vi "Main modul map v3 GPS + kinematyka 2.vi"() -> ()   [LabVIEW 2015]
uses:
  <vilib>/Utility/miscctls.llb/LVPoint32TypeDef.ctl
  Kontrolki/Parametry odwzorowania Ziemi.ctl
  <vilib>/Utility/miscctls.llb/LVBoundsTypeDef.ctl
  <vilib>/Utility/miscctls.llb/LVPointTypeDef.ctl
  <vilib>/Utility/file.llb/Read From Spreadsheet File (string).vi
  Zmienne/szablon odometry_filtered_local.vi
  <vilib>/regexp/Match Regular Expression.xnode
  Pomocnicze/Pomocnicze.lvlib
  Zmienne/Zmienne.lvlib
  Matematyczne/Matematyczne.lvlib
  Kontrolki/Kontrolki.lvlib
panel:
  out "Lokalizacja robotów 2":T1
  in  "stop":bool
  out "Odl. pkt. od startu":cluster{"E/x[m]":dbl, "N/y[m]":dbl}
  out "Numeric":i32
  out "Obr. doj. do pkt.":timestamp
  out "x-y":u32
  in  "Poł. X.":T2={"UTM"={"E [m]"=276177.7293177693, "N [m]"=1172675.379150019, "Strefa"="38P"}, "Piksele"={"X"=991, "Y"=338}} {"UTM"."N [m]" format="%#_10g"}
  out "Mapa":picture caption="Mapa z wprowadzonym punktem"
  out "Lista współrzędnych":string[][](table)
  in  "Tab Control":T3(tab)
  in  "Azymut robota\n pocz/nowy":dbl caption="Azymut robota pocz/nowy" min=0.0 max=360.0
  in  "Lokalizacja mapy terenu":path=path "C:/Users/User/Desktop/Łazik/Mapy do ERL/zoom 19 szarosc - przycieta.jpg"
  in  "Parametry odwzorowania\n Ziemi (WGS84)":T4={"a"=6378137.0, "b"=6356752.3142} {"b" format="%#.6g"; "a" format="%#.6g"}
  in  "Lok. mapy odświeżanej":path=path "C:/Users/User/Desktop/Łazik/Zapis zebranych danych/zapis przejazdu.JPG" caption="Autozapis  mapy terenu"
  in  "Punkt o znanych współrzędnych (X)":T5={"Długość geograficzna - GPS"=10.601698, "Szerokośc geograficzna - GPS"=42.954275} {"Szerokośc geograficzna - GPS" format="%_9f"; "Długość geograficzna - GPS" format="%_9f"}
  in  "Ustawienia początkowe":T6={"Dane z"=TRUE, "Odometria z ROS'a"=TRUE, "GPS"=TRUE, "IMU"=TRUE}
  in  "Zapis danych z przejazdu":T7={"Łazik"=path "C:/Users/User/Desktop/Łazik/Zapis zebranych danych/Łazik.txt", "Quadron"=path "C:/Users/User/Desktop/Łazik/Zapis zebranych danych/Quadron.txt", "Dron 1"=path "C:/Users/User/Desktop/Łazik/Zapis zebranych danych/Dron 1.txt", "Dron 2"=path "C:/Users/User/Desktop/Łazik/Zapis zebranych danych/Dron 2.txt", "Sparus"=path "C:/Users/User/Desktop/Łazik/Zapis zebranych danych/Sparus.txt"}
  in  "Poł. start. robota":bool
  in  "Poł. start. wzgl. bazy":bool
  in  "Zakres skali":u16(ring)=11 items=["OSM 10m", "OSM 30m", "OSM 50m", "OSM 100m", "Google 10m", "Google 50m", "Google 200m1", "Google 100m", "Google 200m 2", "Google 500m", "Google zoom 17", "google zoom 18", "Google zoom 19"]
  in  "Skalowanie":T8={"Polozenie 1"={"X"=265, "Y"=265}, "  Wybór \nznacznika"=FALSE, "   Polozenie 2"={"X"=358, "Y"=265}, "   Blokada \nznaczników"=TRUE, "Kolor  znaczników"=16774930, "Grubość \nznaczników"=2, "Wyznaczanie odległości"=enum."Odległość pomiędzy znacznikami", "Współrzędne geograficzne 1"="", "Współrzędne geograficzne 2"="", "Odl. pomiędzy znacznikami [m]"=15.0}
  in  "Zatwierdz ustalony zakres":bool
  in  "Nazwa akt. pkt":string
  in  "Wpr. pkt. wsp. z pliku":bool
  in  "Plik z punktami wsp. geograficzne":path=path "C:/Users/User/Desktop/ERL 2017/GC.txt"
  in  "Obsługa punktów":T9 {"Usuń punkt z listy"."Punkt do usunięcia" items=["X"=1, "1G"=2, "2G"=3, "3G"=4, "4G"=5, "5G"=6, "6G"=7, "1A"=8, "2A"=9, "3A"=10]}
  in  "Dodaj pkt. poł robota":bool
  in  "Dodaj punkt przed docelowym":u16(ring) items=["X"=1, "1G"=2, "2G"=3, "3G"=4, "4G"=5, "5G"=6, "6G"=7, "1A"=8, "2A"=9, "3A"=10]
  out "Osiągnięcie punktu":bool caption="WP reached"
  out "Punkt\n docelowy":string caption="Punkt  aktualny"
  in  "jazda":bool caption="1. Jazda"
  in  "zad. promien \nodlegl. [m]":dbl=0.3
  in  "2. Autonomia":bool
  in  "Punkt  startowy":u16(ring) items=["X"=1, "1G"=2, "2G"=3, "3G"=4, "4G"=5, "5G"=6, "6G"=7, "1A"=8, "2A"=9, "3A"=10]
  in  "go forward":bool caption="Go forward"
  in  "Time to wait [s]":dbl
  in  "button/time":bool
  in  "Parametry regulatora":cluster{"kp":dbl, "k alfa":dbl, "k beta":dbl}={"kp"=0.2, "k alfa"=0.3, "k beta"=-0.02}
  in  "Dodaj punkt odl.":bool
  in  "Reset":T10
  in  "Wyczyść trasę":bool
  in  "Właściwości mapy":T12={"Przesunięcie mapy"={"X"=0, "Y"=0}, "Dł. px[m]"=0.19634281539316645, "Zoom mapy"=1.0, "Wpisane punkty na\nliście współrzędnych"=1638620, "Zaznaczony punkt"=14417920, "Układ współrzędnych"=786176, "Początkowe położenie robota"=16777215, "Trasa robota - Łazik"=2815743, "Ost. zazn. pkt"={"X"=0, "Y"=0}, "Draw Area Size"={"Width"=528, "Height"=564}} {"Zoom mapy" scale=0.2..6.0}
  out "V - prędkość postępowa":dbl(graph)
  out "w - prędkość kątowa":dbl(graph)
  in  "Wybór robota 3":T13 items=["Łazik", "Quadron", "Dron 1", "Dron 2", "Sparus"]
  in  "Wybór robota 2":T13 items=["Łazik", "Quadron", "Dron 1", "Dron 2", "Sparus"]
  out "Odległości pomiędzy wybranymi robotami xy [m]":cluster{"X [m]":dbl, "Y [m]":dbl}
  out "Odległość pomiędzy\n robotami [m]":dbl
  in  "Wybór robota":T13 items=["Łazik", "Quadron", "Dron 1", "Dron 2", "Sparus"]
  out "Odległość robota  \nod bazy  [m]":cluster{"X [m]":dbl, "Y [m]":dbl}
  out "Azymut":dbl(knob) scale=0.0..360.0
  out "Odczyt GPS":T14 caption="Położenie wybranego robota" {"Szerokośc geograficzna \n- GPS" format="%_9f"; "Długość geograficzna \n- GPS" format="%_9f"; "Położenie \nrobota  UTM"."E [m]" format="%#_10g"; "Położenie \nrobota  UTM"."N [m]" format="%#_12g"}
  in  "Legenda":T15={"Raptor"=16318208, "Quadron"=16711680, "Dron 1"=16777215, "Dron 2"=39423, "Sparus"=6618880}
  in  "Centr. Położenie robota":bool
  in  "Mouse down":T16
  # "Format wprowadzanych współrzędnych:\n0.0d N 0.0d E\n0.0d E 0.0d N\n0d 0.0m N 0d 0.0m E\n0d 0.0m E 0d 0.0m N\n0d 0m 0.0s N 0d 0m 0.0s E\n0d 0m 0.0s E 0d 0m 0.0s N\n\n\"0\" - oznacza dowolny ciąg cyfr. W miejscach gdzie występują liczby\ndziesiętne części całkowite od dziesiętnych są oddzielone znakiem\nkropki \".\".\nd - symbol stopni\nm - symbol minut\ns - symbol sekund\nN - symbol północnej szerokości geograficznej. Dla szerokości geograficznej południowej należy zastosować znak \"S\".\nE - symbol wschodniej długości geograficznej. Dla zachodniej długości geograficznej należy zastosować znak \"W\"."
  # "Nie można usuwać \npunktów, gdy włączona \njest autonomia"
  # "Robot zatrzyma się w najbliższym punkcie,\n który nie zawiera w nazwie litery P"
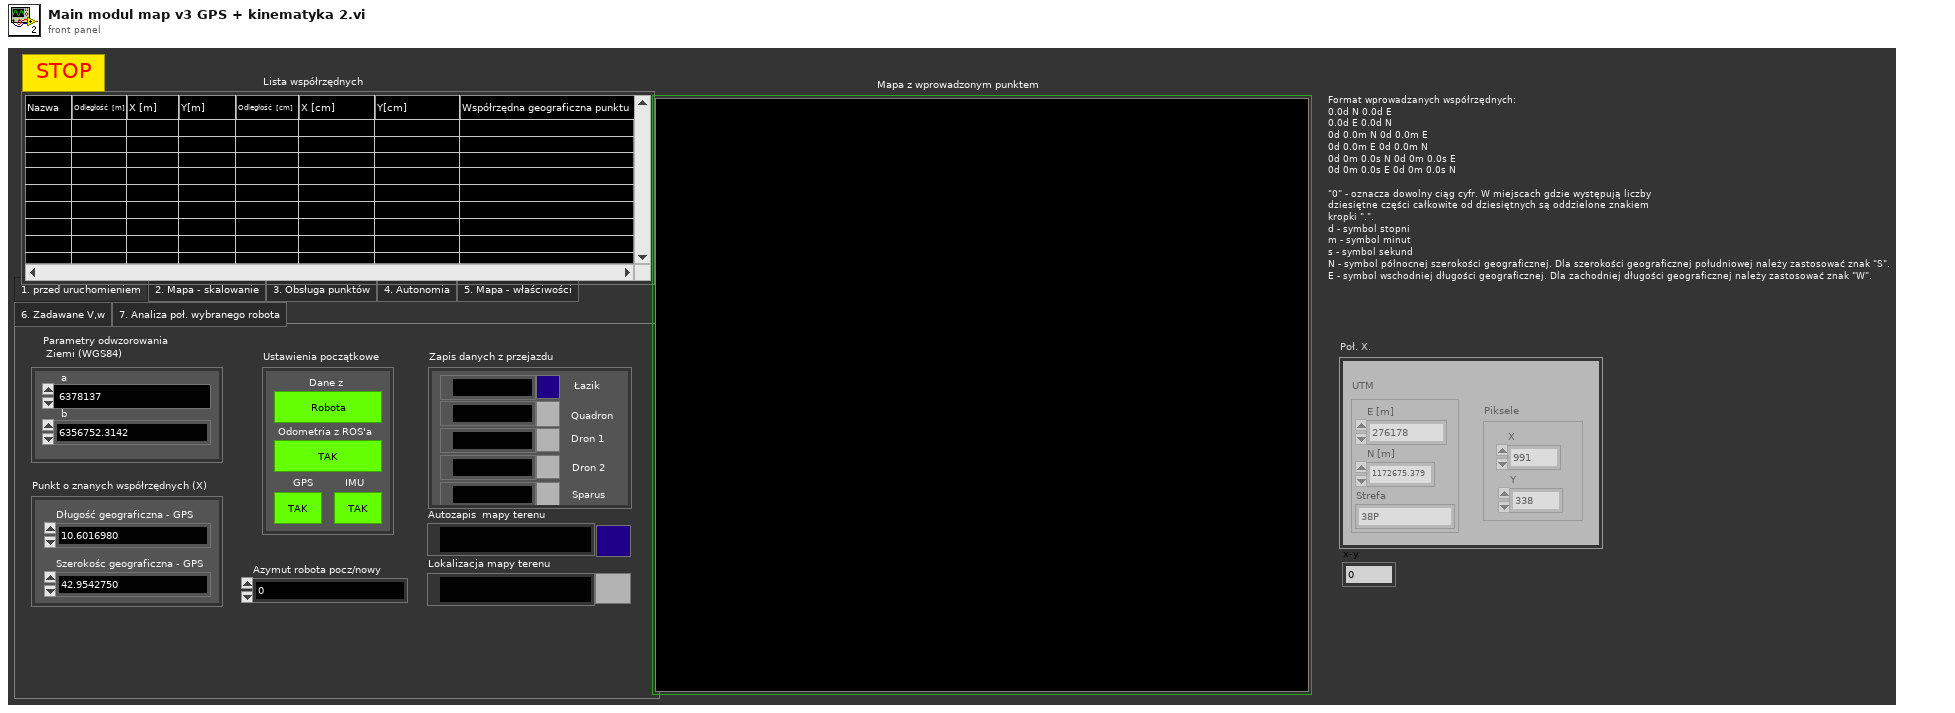
[diagram p1: front panel]
types:
  T1 = typedef "Biblioteka moduł map v3.lvlib/Kontrolki.lvlib/Lokalizacja robotów.ctl" = cluster{"Łazik":cluster{"Odczyt GPS":cluster{"Położenie \nrobota  UTM":cluster{"E [m]":ext, "N [m]":ext, "Strefa":string}, "Długość geograficzna - GPS":dbl, "Szerokośc geograficzna - GPS":dbl, "Azymut [stopnie]":dbl}, "Rzeczywista odległość\n robota od X [m]":cluster{"X [m]":dbl, "Y [m]":dbl}}, "Quadron":cluster{"Odczyt GPS":cluster{"Położenie \nrobota  UTM":cluster{"E [m]":ext, "N [m]":ext, "Strefa":string}, "Długość geograficzna - GPS":dbl, "Szerokośc geograficzna - GPS":dbl, "Azymut [stopnie]":dbl}, "Rzeczywista odległość\n robota od X [m]":cluster{"X [m]":dbl, "Y [m]":dbl}}, "Dron 1":cluster{"Odczyt GPS":cluster{"Położenie \nrobota  UTM":cluster{"E [m]":ext, "N [m]":ext, "Strefa":string}, "Długość geograficzna - GPS":dbl, "Szerokośc geograficzna - GPS":dbl, "Azymut [stopnie]":dbl}, "Rzeczywista odległość\n robota od X [m]":cluster{"X [m]":dbl, "Y [m]":dbl}}, "Dron 2":cluster{"Odczyt GPS":cluster{"Położenie \nrobota  UTM":cluster{"E [m]":ext, "N [m]":ext, "Strefa":string}, "Długość geograficzna - GPS":dbl, "Szerokośc geograficzna - GPS":dbl, "Azymut [stopnie]":dbl}, "Rzeczywista odległość\n robota od X [m]":cluster{"X [m]":dbl, "Y [m]":dbl}}, "Sparus":cluster{"Odczyt GPS":cluster{"Położenie \nrobota  UTM":cluster{"E [m]":ext, "N [m]":ext, "Strefa":string}, "Długość geograficzna - GPS":dbl, "Szerokośc geograficzna - GPS":dbl, "Azymut [stopnie]":dbl}, "Rzeczywista odległość\n robota od X [m]":cluster{"X [m]":dbl, "Y [m]":dbl}}}
  T2 = cluster{"UTM":cluster{"E [m]":dbl, "N [m]":dbl, "Strefa":string}, "Piksele":cluster{"X":i32, "Y":i32}}
  T3 = enum32{"1. przed uruchomieniem", "2. Mapa - skalowanie", "3. Obsługa punktów", "4. Autonomia", "5. Mapa - właściwości", "6. Zadawane V,w", "7. Analiza poł. wybranego robota"}
  T4 = typedef "Biblioteka moduł map v3.lvlib/Kontrolki.lvlib/Parametry odwzorowania Ziemi.ctl" = cluster{"a":dbl, "b":dbl}
  T5 = cluster{"Długość geograficzna - GPS":dbl, "Szerokośc geograficzna - GPS":dbl}
  T6 = cluster{"Dane z":bool, "Odometria z ROS'a":bool, "GPS":bool, "IMU":bool}
  T7 = cluster{"Łazik":path, "Quadron":path, "Dron 1":path, "Dron 2":path, "Sparus":path}
  T8 = cluster{"Polozenie 1":cluster{"X":i32, "Y":i32}, "  Wybór \nznacznika":bool, "   Polozenie 2":cluster{"X":i32, "Y":i32}, "   Blokada \nznaczników":bool, "Kolor  znaczników":u32, "Grubość \nznaczników":u32, "Wyznaczanie odległości":enum16{"Współrzędne geograficzne", "Odległość pomiędzy znacznikami"}, "Współrzędne geograficzne 1":string, "Współrzędne geograficzne 2":string, "Odl. pomiędzy znacznikami [m]":dbl}
  T9 = cluster{"Zaznaczony punkt":cluster{"Nazwa":string, "Odl. do pkt [m]":cluster{"X":dbl, "Y":dbl}, "Dodaj punkt odl.":bool}, "Wsp. geograficzne":cluster{"Nazwa":string, "Współrzędna punktu":string, "Dodaj punkt wsp.":bool}, "Usuń punkt z listy":cluster{"Punkt do usunięcia":u16, "Usuń punkt":bool}}
  T10 = cluster{"reset odom":bool, "reset odom + gps":bool}
  T11 = typedef "LVBoundsTypeDef.ctl" = cluster{"Width":u32, "Height":u32}
  T12 = cluster{"Przesunięcie mapy":cluster{"X":i16, "Y":i16}, "Dł. px[m]":dbl, "Zoom mapy":sgl, "Wpisane punkty na\nliście współrzędnych":u32, "Zaznaczony punkt":u32, "Układ współrzędnych":u32, "Początkowe położenie robota":u32, "Trasa robota - Łazik":u32, "Ost. zazn. pkt":cluster{"X":i32, "Y":i32}, "Draw Area Size":T11}
  T13 = typedef "Biblioteka moduł map v3.lvlib/Kontrolki.lvlib/Wybór robota.ctl" = u16
  T14 = cluster{"Położenie \nrobota  UTM":cluster{"E [m]":ext, "N [m]":ext, "Strefa":string}, "Długość geograficzna \n- GPS":dbl, "Szerokośc geograficzna \n- GPS":dbl, "Azymut [stopnie]":dbl}
  T15 = cluster{"Raptor":u32, "Quadron":u32, "Dron 1":u32, "Dron 2":u32, "Sparus":u32}
  T16 = typedef "LVPoint32TypeDef.ctl" = cluster{"Horizontal":i32, "Vertical":i32}
  T17 = enum16{"Pobranie punktu", "Obrót i dojazd do punktu", "Zatrzymanie w punkcie"}
  T18 = cluster{"UTM":cluster{"E [m]":ext, "N [m]":ext, "Strefa":string}, "Piksele":cluster{"X":i32, "Y":i32}}
  T19 = typedef "Biblioteka moduł map v3.lvlib/Zmienne.lvlib/szablon odometry_filtered_local.ctl" = cluster{"topic":string, "msg":cluster{"header":cluster{"seq":u32, "stamp":cluster{"secs":u32, "nsecs":i32}, "frame_id":string}, "child_frame_id":string, "pose":cluster{"pose":cluster{"position":cluster{"y":dbl, "z":dbl, "x":dbl}, "orientation":cluster{"y":dbl, "z":dbl, "x":dbl, "w":dbl}}, "covariance":dbl[]}, "twist":cluster{"twist":cluster{"linear":cluster{"y":dbl, "z":dbl, "x":dbl}, "angular":cluster{"y":dbl, "z":dbl, "x":dbl}}, "covariance":dbl[]}}, "op":string}
  T20 = cluster{"left":i16, "top":i16, "right":i16, "bottom":i16}
  T21 = cluster{"Nazwa zaznaczonego punktu":string, "Odleglosc do\n zaznaczonego punktu [m]":cluster{"X":dbl, "Y":dbl}}
  T22 = cluster{"Kolor punktów z listy":u32, "Położenie startowe robota":cluster{"Pixel y":i16, "Pixel x":i16}}
  T23 = typedef "LVPointTypeDef.ctl" = cluster{"Horizontal":i16, "Vertical":i16}
  T24 = cluster{"E [m]":dbl, "N [m]":dbl, "Strefa":string}
  T25 = typedef "LVMouseTypeDef.ctl" = cluster{"Mouse Position":cluster{"X":i32, "Y":i32}, "Mouse Modifiers":cluster{"Button Down":bool, "Shift Mod":bool, "Menu Mod":bool, "Option Mod":bool}}
  T26 = cluster{"Przesunięcie mapy":cluster{"X":i16, "Y":i16}, "Długość piksela w metrach":dbl, "Zoom mapy":sgl, "Wpisane punkty na\nliście współrzędnych":u32, "Zaznaczony punkt":u32, "Układ współrzędnych":u32, "Początkowe położenie robota":u32, "Trasa robota":u32, "Ost. zazn. pkt.":cluster{"X":i32, "Y":i32}, "Draw Area Size":T11}
  T27 = cluster{"Zaznaczony punkt":cluster{"Nazwa":string, "Odleglosc do\n zaznaczonego punktu [m]":cluster{"X":dbl, "Y":dbl}, "Dodaj punkt odl.":bool}, "Wsp. geograficzne":cluster{"Nazwa":string, "Współrzędna punktu":string, "Dodaj punkt wsp.":bool}, "Usuń punkt z listy":cluster{"Punkt do usunięcia":u16, "Usuń punkt":bool}}
  T28 = cluster{"E [m]":ext, "N [m]":ext, "Strefa":string}
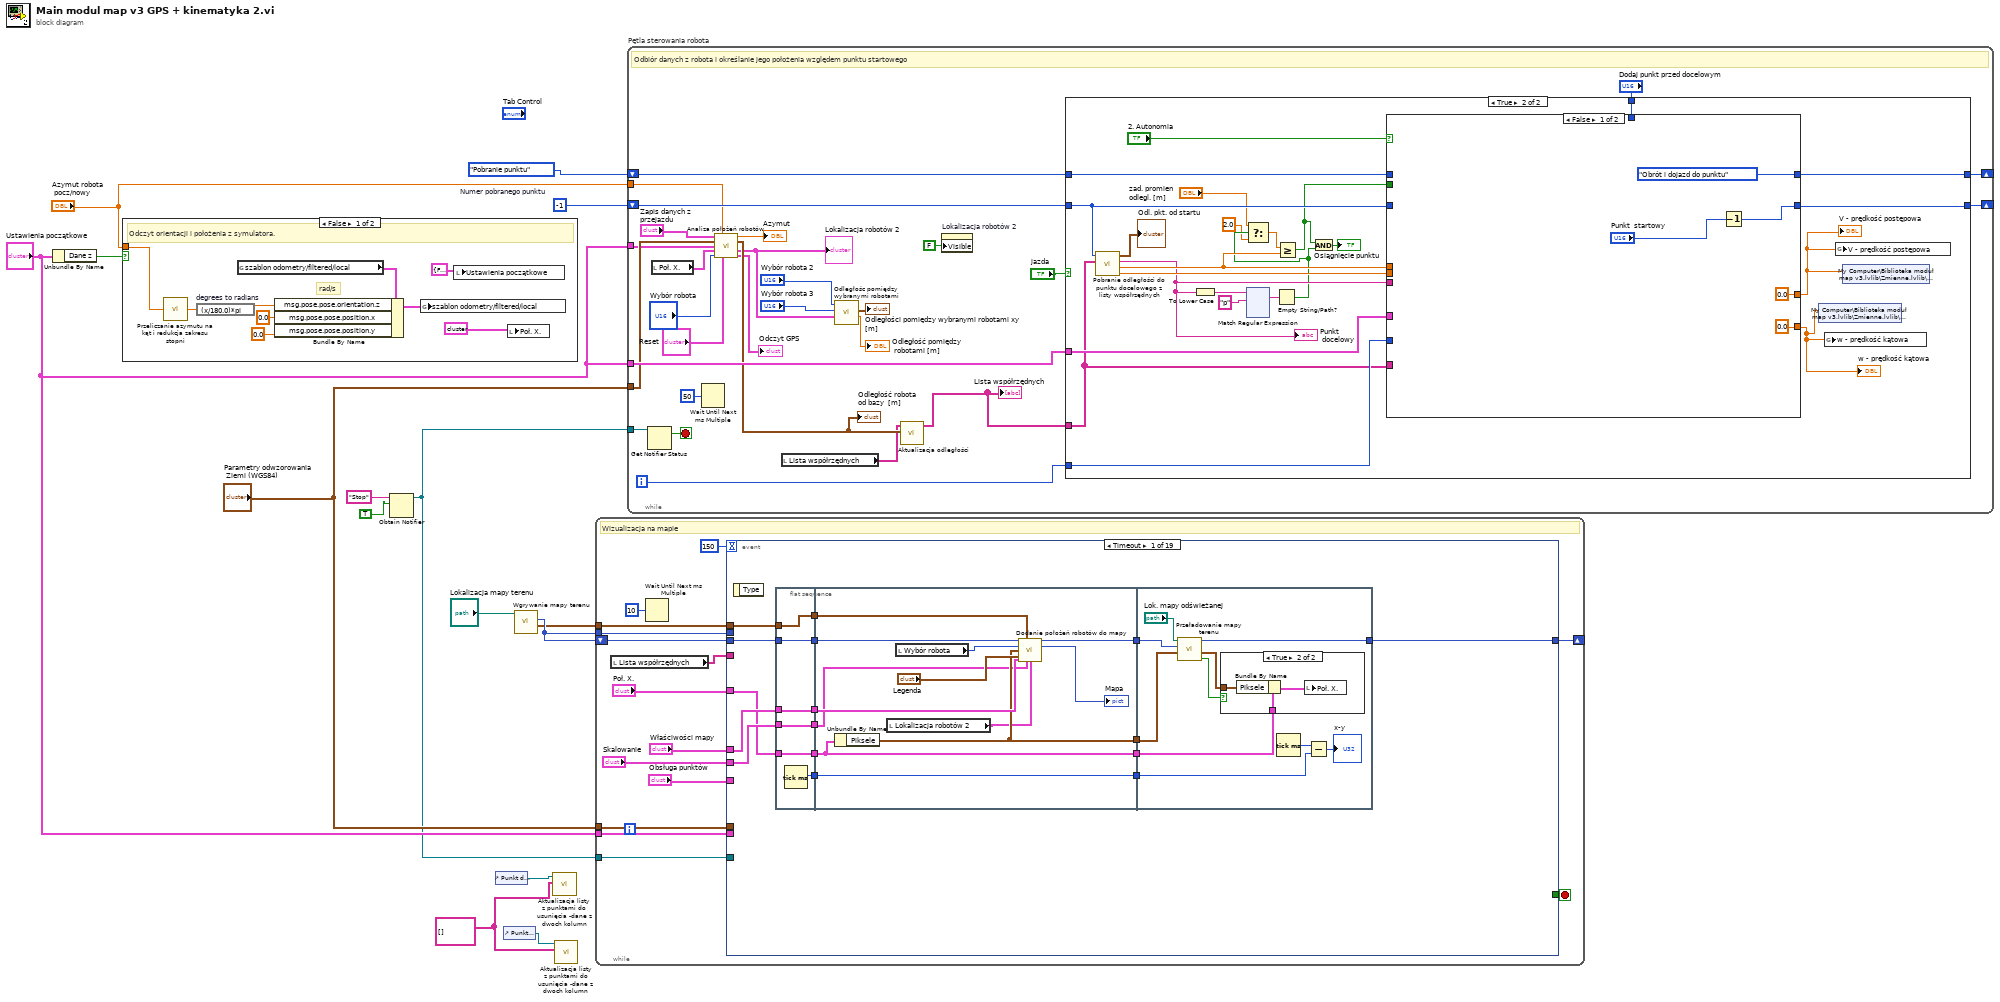
[diagram p0: block diagram]
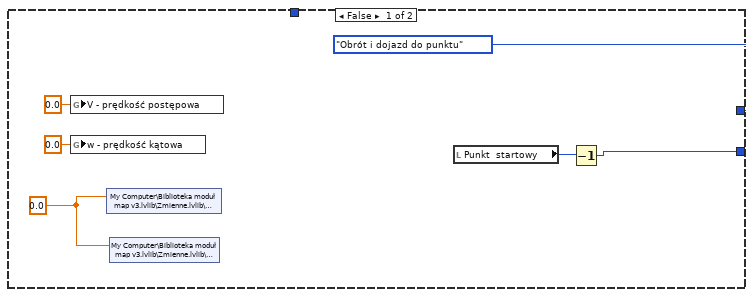
[diagram p3: hidden frame]
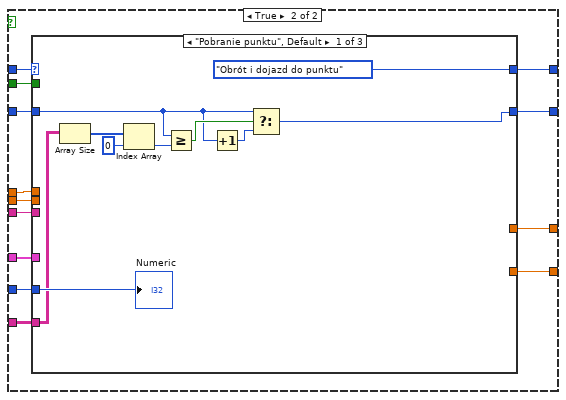
[diagram p4: hidden frame]
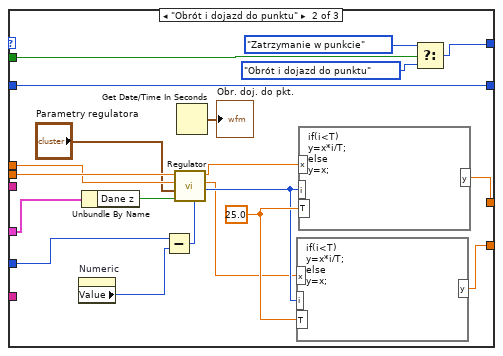
[diagram p5: hidden frame]
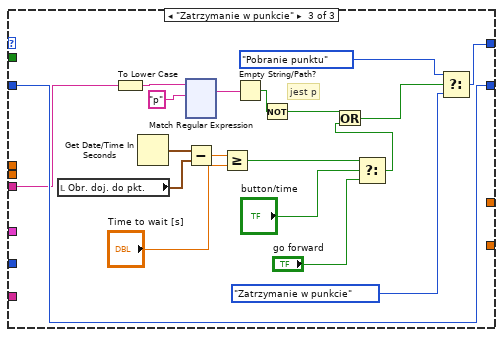
[diagram p6: hidden frame]
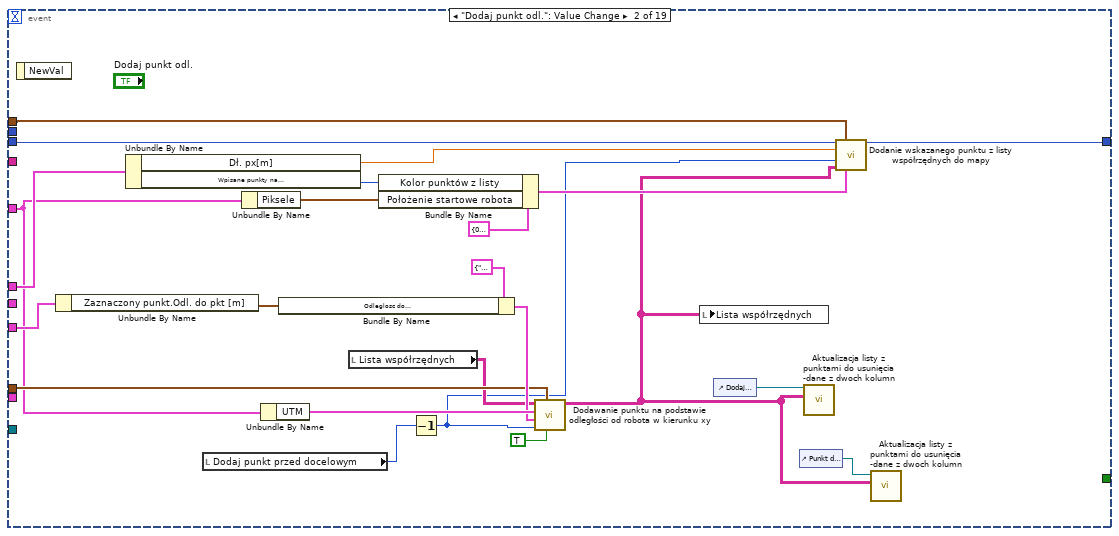
[diagram p8: hidden frame]
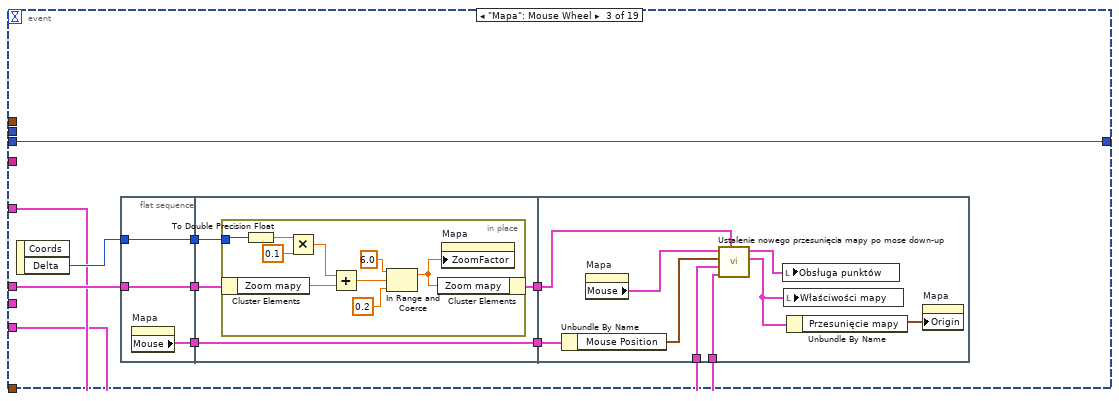
[diagram p9: hidden frame]
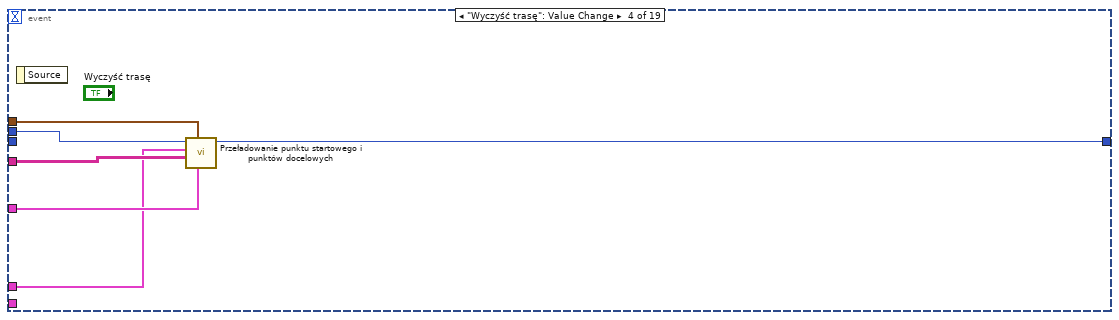
[diagram p10: hidden frame]
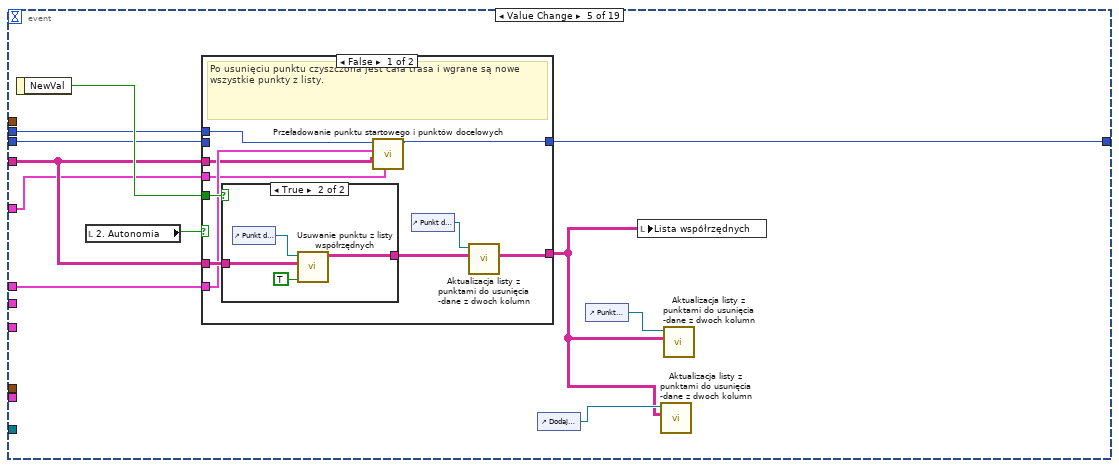
[diagram p11: hidden frame]
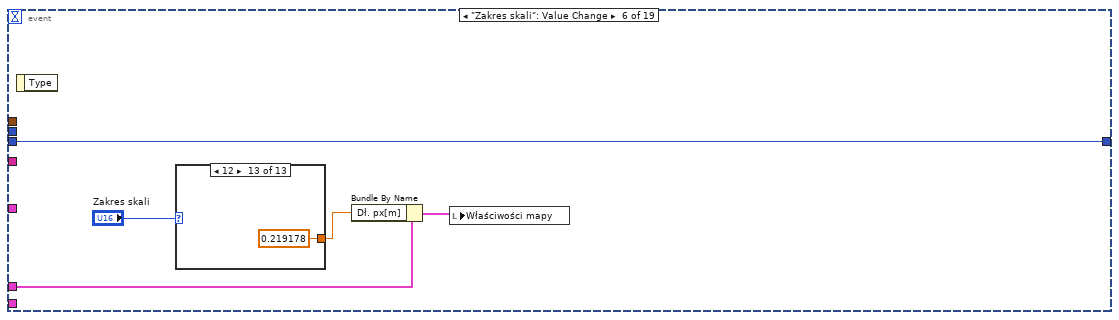
[diagram p14: hidden frame]
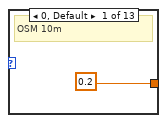
[diagram p15: hidden frame]
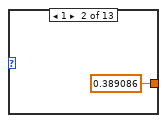
[diagram p16: hidden frame]
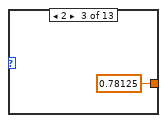
[diagram p17: hidden frame]
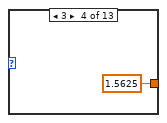
[diagram p18: hidden frame]
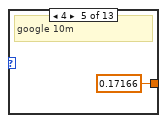
[diagram p19: hidden frame]
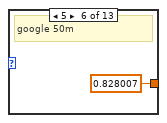
[diagram p20: hidden frame]
diagram:
  w5 = string[][] [] ("Lista współrzędnych")
  w14 = -1  # Numer pobranego punktu
  n1 = Unbundle By Name("Ustawienia początkowe") -> ("Dane z"=w4:bool)
  n2 = case shown="False" w4 {
    tunnel: "Azymut robota\n pocz/nowy" -> [w17 _]
    frame False {
      # "rad/s"
      # "Odczyt orientacji i położenia z symulatora."
      n3 = call "Przeliczanie azymutu na kąt i redukcja zakresu stopni.vi"("Azymut [stoponie]"=w17) -> ("Kąt [stopnie]"=w19:dbl)  [unwired: 4 in]
      n4 = expression code="(x/180.0)*pi" "degrees to radians"(w19) -> (w22:dbl)
      n5 = global read "szablon odometry_filtered_local.vi" "szablon odometry/filtered/local"() -> (w24:T19)
      n6 = Bundle By Name(cluster=w24, "msg.pose.pose.orientation.z"=w22, "msg.pose.pose.position.x"=0.0, "msg.pose.pose.position.y"=0.0) -> (w23:T19)
      n7 = global write "szablon odometry_filtered_local.vi" "szablon odometry/filtered/local"(w23) -> ()
      n8 = local write "Ustawienia początkowe"(T6 {"Dane z"=FALSE, "Odometria z ROS'a"=FALSE, "GPS"=FALSE, "IMU"=FALSE} ("Ustawienia początkowe")) -> ()
      n9 = local write "Poł. X."(T18 {"UTM"={"E [m]"=0.0, "N [m]"=0.0, "Strefa"=""}, "Piksele"={"X"=0, "Y"=0}} ("Pocz. bazowe.")) -> ()
    }
    frame True {
      # "Dane odczytywane z robota i zapisane w zmiennej globalnej."
    }
  }
  n10 = Obtain Notifier(name (unnamed)="Stop", notification data type=TRUE ("create if not found? (T)")) -> (notifier out=w1:refnum<notifier>)  [unwired: 2 in, 2 out]
  n11 = control-ref of="Punkt do usunięcia"() -> (w8:refnum<vi>)
  n12 = control-ref of="Punkt  startowy"() -> (w7:refnum<vi>)
  n13 = call "Wgrywanie mapy terenu.vi"("Lokalizacja mapy terenu"="Lokalizacja mapy terenu") -> ("Rozmiar mapy"=w6:T20, "Mapa terenu"=w12:picture)  [unwired: 9 in]
  n14 = call "Aktualizacja listy z punktami do usunięcia -dane z dwoch kolumn.vi"("Lista współrzędnych"=w5, "Lista z punktami do usunięcia"=w8) -> ()  [unwired: 10 in]
  n15 = call "Aktualizacja listy z punktami do usunięcia -dane z dwoch kolumn.vi"("Lista współrzędnych"=w5, "Lista z punktami do usunięcia"=w7) -> ()  [unwired: 10 in]
  n16 = while "Pętla obsługi mapy" {
    shift-right: [w36] -> _
    shift-left: w12 -> [w37]
    tunnel: "Parametry odwzorowania\n Ziemi (WGS84)" -> [w35]
    tunnel: w1 -> [w34]
    tunnel: w12 -> [w30]
    tunnel: w6 -> [w28]
    tunnel: "Ustawienia początkowe" -> [w27]
    stop <- w39 stop-if-true
    # "Wizualizacja na mapie"
    n17 = local read "Lista współrzędnych"() -> (w25:string[][])
    n18 = Wait Until Next ms Multiple(millisecond multiple=u32 10) -> ()  [unwired: 1 out]
    n19 = event shown="[0] Timeout" {
      selector: _ -> [_ _ _ _ _ _ _ _ _ _ _ _ _ _ _ _ _ _ _]
      dyn-events: _ -> [_ _ _ _ _ _ _ _ _ _ _ _ _ _ _ _ _ _ _]
      timeout: 150 -> [_ _ _ _ _ _ _ _ _ _ _ _ _ _ _ _ _ _ _]
      tunnel: "Właściwości mapy" -> [w54 w102 w117 w146 w155 w181 w213 w280 w292 w298 w315 w330 w351 w369 _ w386 w404 w430 w451]
      tunnel: w37 -> [w52 w103 w119 _ w157 w182 w216 w274 _ _ w321 w331 _ w371 w374 w387 w401 w437 w446]
      tunnel: [_ _ _ _ _ _ _ _ _ _ _ _ _ w365 _ _ _ _ _] -> w39
      tunnel: [w51 w101 w119 w150 w158 w182 w215 w272 w288 w299 w321 w331 w352 w371 w374 w387 w405 w437 w443] -> w36
      tunnel: w25 -> [_ _ _ w147 w154 _ w202 w282 w289 w301 _ _ w356 _ _ _ w408 _ w460]
      tunnel: w35 -> [_ w95 _ _ _ _ _ w285 _ w303 _ _ _ _ _ _ _ _ _]
      tunnel: w34 -> [_ _ _ _ _ _ _ _ _ _ _ _ _ w370 _ _ _ _ _]
      tunnel: "Poł. X." -> [w50 w94 w113 w148 w153 _ w209 w271 w286 _ _ w327 w344 _ _ w375 w403 w423 w442]
      tunnel: "Skalowanie" -> [w53 _ _ _ _ _ _ _ w295 _ _ _ _ _ _ w377 _ _ _]
      tunnel: "Obsługa punktów" -> [_ w96 w112 _ _ _ _ w283 _ _ _ _ _ _ _ w384 _ w426 w455]
      tunnel: w30 -> [_ _ _ w149 w156 _ _ _ w291 w302 _ _ w355 _ _ _ _ _ _]
      tunnel: w28 -> [w41 w104 _ w145 _ _ w214 w269 w287 w297 _ w323 w350 _ _ _ w400 _ w440]
      tunnel: w27 -> [_ _ _ _ _ _ w199 _ _ w300 _ _ w354 _ _ _ _ _ _]
      event Timeout {
        n20 = event-data() -> ()  [unwired: 1 in, 1 out]
        n21 = flat-sequence {
          tunnel: w50 -> [w58]
          tunnel: w52 -> [w59]
          tunnel: w53 -> [w60]
          tunnel: w54 -> [w61]
          tunnel: [w61] -> w47
          tunnel: [w60] -> w46
          tunnel: [w59] -> w45
          tunnel: [w58] -> w44
          tunnel: [w57] -> w43
          tunnel: w41 -> [w56]
          tunnel: [w56] -> w40
          tunnel: [w70] -> w55
          tunnel: [w64] -> w49
          tunnel: [w73] -> w48
          tunnel: w47 -> [w65]
          tunnel: w46 -> [w62]
          tunnel: w45 -> [w69]
          tunnel: w44 -> [w73]
          tunnel: w43 -> [w72]
          tunnel: [w72] -> w42
          tunnel: w40 -> [w68]
          tunnel: [w83] -> w51
          tunnel: w55 -> [w82]
          tunnel: w49 -> [w74]
          tunnel: w48 -> [w78]
          tunnel: w42 -> [w76]
          frame #0 {
            n22 = Tick Count (ms)() -> (millisecond timer value=w57:u32)
          }
          frame #1 {
            n23 = Unbundle By Name(w73) -> ("Piksele"=w64:cluster{"X":i32, "Y":i32})
            n24 = local read "Lokalizacja robotów 2"() -> (w63:T1)
            n25 = local read "Wybór robota"() -> (w67:T13)
            n26 = call "Dodanie położeń robotów do mapy.vi"("Mapa terenu"=w69, "Rozmiar mapy"=w68, "Wybór robota"=w67, "Poł. bazowe\n piksele"=w64, "Właściwości mapy"=w65, "Skalowanie i kolory"=w62, "Lokalizacja robotów"=w63, "Legenda"="Legenda") -> ("Mapa terenu stała"=w70:picture, "Mapa terenu wyświetlana"=→"Mapa":picture)  [unwired: 6 in]
          }
          frame #2 {
            n27 = call "Przeładowanie mapy terenu.vi"("Położenie startowe"=w74, ">mapa z trasą robota>"=w82, "path to JPEG file"="Lok. mapy odświeżanej") -> ("reload"=w81:bool, "Nowe położenie  startowe [px]"=w79:cluster{"X [px]":i16, "Y [px]":i16}, "Mapa terenu"=w83:picture)  [unwired: 6 in]
            n28 = case shown="True" w81 {
              tunnel: w79 -> [_ w86]
              tunnel: w78 -> [_ w85]
              frame False {
              }
              frame True {
                n29 = Bundle By Name(cluster=w85, "Piksele"=w86) -> (w84:T2)
                n30 = local write "Poł. X."(w84) -> ()
              }
            }
            n31 = Tick Count (ms)() -> (millisecond timer value=w77:u32)
            n32 = Subtract(x=w77, y=w76) -> (x-y=→"x-y":u32)
          }
        }
      }
      event "Dodaj punkt odl.": Value Change {
        n33 = event-data() -> ()  [unwired: 1 in, 1 out]
        n34 = Unbundle By Name(w96) -> ("Zaznaczony punkt.Odl. do pkt [m]"=w100:cluster{"X":dbl, "Y":dbl})
        n35 = Unbundle By Name(w102) -> ("Dł. px[m]"=w107:dbl, "Wpisane punkty na\nliście współrzędnych"=w108:u32)
        n36 = local read "Dodaj punkt przed docelowym"() -> (w88:u16)
        n37 = Unbundle By Name(w94) -> ("Piksele"=w105:cluster{"X":i32, "Y":i32})
        n38 = Unbundle By Name(w94) -> ("UTM"=w99:T24)
        n39 = Bundle By Name(cluster=T21 {"Nazwa zaznaczonego punktu"="p ", "Odleglosc do\n zaznaczonego punktu [m]"={"X"=23.89186471933565, "Y"=43.80175198544869}} ("Zaznaczony punkt"), "Odleglosc do\n zaznaczonego punktu [m]"=w100) -> (w98:T21)
        n40 = local read "Lista współrzędnych"() -> (w89:string[][])
        n41 = Bundle By Name(cluster=T22 {"Kolor punktów z listy"=0, "Położenie startowe robota"={"Pixel y"=0, "Pixel x"=0}} ("Właściwości punktów z listy"), "Kolor punktów z listy"=w108, "Położenie startowe robota"=w105) -> (w106:T22)
        n42 = Decrement(x=w88) -> (x-1=w87:u16)
        n43 = call "Dodawanie punktu na podstawie odległości od robota w kierunku xy.vi"("dodanie posredniego punktu w trybie autonomi"=TRUE, "Parametry odwzorowania Ziemi"=w95, "Nr wiersza do wpisania punktu"=w87, "Zaznaczony punkt"=w98, "Początkowe UTM"=w99, "Lista współrzędnych"=w89) -> ("output array"=w90:string[][])  [unwired: 5 in]
        n44 = local write "Lista współrzędnych"(w90) -> ()
        n45 = control-ref of="Dodaj punkt przed docelowym"() -> (w91:refnum<vi>)
        n46 = control-ref of="Punkt do usunięcia"() -> (w92:refnum<vi>)
        n47 = call "Aktualizacja listy z punktami do usunięcia -dane z dwoch kolumn.vi"("Lista współrzędnych"=w90, "Lista z punktami do usunięcia"=w91) -> ()  [unwired: 10 in]
        n48 = call "Dodanie wskazanego punktu z listy współrzędnych do mapy.vi"("Mapa terenu"=w103, "Rozmiar mapy"=w104, "Długość piksela w metrach"=w107, "Nr punktu"=w87, "Lista współrzędnych"=w90, "Właściwości punktów z listy"=w106) -> ("Mapa z wprowadzonym punktem"=w101:picture)  [unwired: 9 in]
        n49 = call "Aktualizacja listy z punktami do usunięcia -dane z dwoch kolumn.vi"("Lista współrzędnych"=w90, "Lista z punktami do usunięcia"=w92) -> ()  [unwired: 10 in]
      }
      event "Mapa": Mouse Wheel {
        n50 = event-data() -> ("Delta"=w118:i32)  [unwired: 1 in, 1 out]
        n51 = flat-sequence {
          tunnel: w117 -> [w121]
          tunnel: w118 -> [w122]
          tunnel: [w122] -> w116
          tunnel: [w121] -> w115
          tunnel: [w120] -> w111
          tunnel: w116 -> [w126]
          tunnel: w115 -> [w125]
          tunnel: [w124] -> w114
          tunnel: w111 -> [w123]
          tunnel: [w123] -> w110
          tunnel: w114 -> [w137]
          tunnel: w113 -> [w140]
          tunnel: w112 -> [w139]
          tunnel: w110 -> [w136]
          frame #0 {
            n52 = property on="Mapa" class="Pict"() -> ("Mouse"=w120:T25)  [unwired: 2 in, 2 out]
          }
          frame #1 {
            n53 = in-place {
              in-place-border: w126 -> [w134]
              n54 = in-place-cluster #1(w125) -> ("Zoom mapy"=w131:sgl)
              n55 = To Double Precision Float(number=w134) -> (double precision float=w135:dbl)
              n56 = Multiply(x=w135, y=0.1) -> (x*y=w132:dbl)
              n57 = Add(x=w132, y=w131) -> (x+y=w130:dbl)
              n58 = In Range and Coerce(upper limit=6.0, x=w130, lower limit=0.2) -> (coerced(x)=w127:dbl)  [unwired: 1 out]
              n59 = in-place-cluster #1("Zoom mapy"=w127) -> (w124:T12)
              n60 = property on="Mapa" class="Pict"("ZoomFactor"=w127) -> ()  [unwired: 2 in, 2 out]
            }
          }
          frame #2 {
            n61 = Unbundle By Name(w136) -> ("Mouse Position"=w144:cluster{"X":i32, "Y":i32})
            n62 = property on="Mapa" class="Pict"() -> ("Mouse"=w138:T25)  [unwired: 2 in, 2 out]
            n63 = call "Ustalenie nowego przesunięcia mapy po mose down-up.vi"("Właściwości mapy in"=w137, "Pocz. poł."=w140, "Obsługa punktów in"=w139, "Mouse down \ncoords"=w144, "Mouse"=w138) -> ("Właściwości mapy out"=w142:T26, "Obsługa punktów out"=w141:T27)  [unwired: 5 in]
            n64 = local write "Obsługa punktów"(w141) -> ()
            n65 = local write "Właściwości mapy"(w142) -> ()
            n66 = Unbundle By Name(w142) -> ("Przesunięcie mapy"=w143:cluster{"X":i16, "Y":i16})
            n67 = property on="Mapa" class="Pict"("Origin"=w143) -> ()  [unwired: 2 in, 2 out]
          }
        }
      }
      event "Wyczyść trasę": Value Change {
        n68 = event-data() -> ()  [unwired: 1 in, 1 out]
        n69 = call "Przeładowanie punktu startowego i punktów docelowych.vi"("Pocz. poł. startu"=w148, "Rozmiar mapy"=w145, "Lista współrzędnych"=w147, "Właściwości mapy"=w146, "Mapa terenu"=w149) -> ("Mapa z wprowadzonym punktem"=w150:picture)  [unwired: 6 in]
      }
      event "Obsługa punktów.Usuń punkt z listy.Usuń punkt": Value Change {
        n70 = event-data() -> ("NewVal"=w161:bool)  [unwired: 1 in]
        n71 = local read "2. Autonomia"() -> (w160:bool)
        n72 = case shown="False" w160 {
          tunnel: w161 -> [w170 _]
          tunnel: w154 -> [w168 w177]
          tunnel: [w167 w177] -> w151
          tunnel: w157 -> [_ w176]
          tunnel: [w166 w176] -> w158
          tunnel: w156 -> [w165 _]
          tunnel: w155 -> [w164 _]
          tunnel: w154 -> [w163 _]
          tunnel: w153 -> [w162 _]
          frame False {
            # "Po usunięciu punktu czyszczona jest cała trasa i wgrane są nowe wszystkie punkty z listy."
            n73 = case shown="True" w170 {
              tunnel: w168 -> [w171 w174]
              tunnel: [w171 w173] -> w167
              frame False {
              }
              frame True {
                n74 = control-ref of="Punkt do usunięcia"() -> (w175:refnum<vi>)
                n75 = call "Usuwanie punktu z listy współrzędnych.vi"("Aktywacja potwierdzenia"=TRUE, "Lista współrzędnych"=w174, "Lista z punktami do usunięcia"=w175) -> ("Lista współrzędnych 2"=w173:string[][])  [unwired: 8 in]
              }
            }
            n76 = call "Przeładowanie punktu startowego i punktów docelowych.vi"("Pocz. poł. startu"=w162, "Lista współrzędnych"=w163, "Właściwości mapy"=w164, "Mapa terenu"=w165) -> ("Mapa z wprowadzonym punktem"=w166:picture)  [unwired: 7 in]
            n77 = control-ref of="Punkt do usunięcia"() -> (w169:refnum<vi>)
            n78 = call "Aktualizacja listy z punktami do usunięcia -dane z dwoch kolumn.vi"("Lista współrzędnych"=w167, "Lista z punktami do usunięcia"=w169) -> ()  [unwired: 10 in]
          }
          frame True {
          }
        }
        n79 = control-ref of="Dodaj punkt przed docelowym"() -> (w152:refnum<vi>)
        n80 = control-ref of="Punkt  startowy"() -> (w159:refnum<vi>)
        n81 = local write "Lista współrzędnych"(w151) -> ()
        n82 = call "Aktualizacja listy z punktami do usunięcia -dane z dwoch kolumn.vi"("Lista współrzędnych"=w151, "Lista z punktami do usunięcia"=w152) -> ()  [unwired: 10 in]
        n83 = call "Aktualizacja listy z punktami do usunięcia -dane z dwoch kolumn.vi"("Lista współrzędnych"=w151, "Lista z punktami do usunięcia"=w159) -> ()  [unwired: 10 in]
      }
      event "Zakres skali": Value Change {
        n84 = event-data() -> ()  [unwired: 1 in, 1 out]
        n85 = case shown="12" "Zakres skali" {
          tunnel: [0.2 0.389086 0.78125 1.5625 0.17166 0.828007 4.25179 3.81711 2.13015 8.47336 0.943026 0.471513 0.219178] -> w179
          frame 0, Default {
            # "OSM 10m"
          }
          frame 1 {
          }
          frame 2 {
          }
          frame 3 {
          }
          frame 4 {
            # "google 10m"
          }
          frame 5 {
            # "google 50m"
          }
          frame 6 {
            # "200m1"
          }
          frame 7 {
            # "100m"
          }
          frame 8 {
            # "200m2"
          }
          frame 9 {
            # "500m popr."
          }
          frame 10 {
            # "zoom 17 MPuzle"
          }
          frame 11 {
            # "18 zoom MP"
          }
          frame 12 {
          }
        }
        n86 = Bundle By Name(cluster=w181, "Dł. px[m]"=w179) -> (w180:T12)
        n87 = local write "Właściwości mapy"(w180) -> ()
      }
      event "Dodaj pkt. poł robota": Value Change {
        n88 = event-data() -> ()  [unwired: 1 in, 1 out]
        n89 = Unbundle By Name(w199) -> ("GPS"=w198:bool)
        n90 = Unbundle By Name(w209) -> ("Piksele"=w208:cluster{"X":i32, "Y":i32})
        n91 = Unbundle By Name(w213) -> ("Dł. px[m]"=w212:dbl, "Wpisane punkty na\nliście współrzędnych"=w207:u32)
        n92 = case shown="True" w198 {
          tunnel: [w237 w264] -> w196
          tunnel: w202 -> [w229 w263]
          tunnel: w209 -> [_ w262]
          tunnel: "Nazwa akt. pkt" -> [w222 w248]
          frame False {
            w224 = ""
            n93 = Array Size(array=w229) -> (size(s)=w235:i32[])
            n94 = local read "Odległość robota  \nod bazy  [m]"() -> (w217:cluster{"X [m]":dbl, "Y [m]":dbl})
            n95 = Index Array(array=w235, index=0) -> (element=w233:i32)
            n96 = Equal?(x=w222, y="Start") -> (x = y?=w221:bool)
            n97 = Increment(x=w233) -> (x+1=w232:i32)
            n98 = Number To Decimal String(number=w232) -> (decimal integer string=w230:string)  [unwired: 1 in]
            n99 = Empty String/Path?(string/path=w222) -> (empty?=w231:bool)
            n100 = Select(t=w230, s=w231, f=w222) -> (s? t:f=w220:string)
            n101 = Unbundle By Name(w217) -> ("X [m]"=w228:dbl, "Y [m]"=w227:dbl)
            n102 = Select(t="", s=w221, f=w220) -> (s? t:f=w219:string)
            n103 = Number To Fractional String(number=w228) -> (F-format string=w226:string)  [unwired: 3 in]
            n104 = Number To Fractional String(number=w227) -> (F-format string=w225:string)  [unwired: 3 in]
            n105 = Build Array(w219, w224, w224, w224, w224, w224, w224, w224, w224, w224, w224, w226, w225) -> (w236:string[])
            n106 = Insert Into Array(array=w229, new element=w236) -> (w237:string[][])  [unwired: 2 in]
          }
          frame True {
            n107 = local read "Odczyt GPS"() -> (w240:T14)
            n108 = Unbundle By Name(w262) -> ("UTM"=w261:T24)
            n109 = Unbundle By Name(w240) -> ("Długość geograficzna \n- GPS"=w239:dbl, "Szerokośc geograficzna \n- GPS"=w238:dbl)
            n110 = Greater Or Equal To 0?(x=w238) -> (x >= 0?=w258:bool)
            n111 = Absolute Value(x=w239) -> (abs(x)=w259:dbl)
            n112 = Greater Or Equal To 0?(x=w239) -> (x >= 0?=w257:bool)
            n113 = Absolute Value(x=w238) -> (abs(x)=w260:dbl)
            n114 = Number To Fractional String(number=w259) -> (F-format string=w252:string)  [unwired: 3 in]
            n115 = Select(t="d N " ("f"), s=w258, f="d S ") -> (s? t:f=w249:string)
            n116 = Number To Fractional String(number=w260) -> (F-format string=w250:string)  [unwired: 3 in]
            n117 = Select(t="d E " ("f"), s=w257, f="d W ") -> (s? t:f=w251:string)
            n118 = Concatenate Strings(w252, w251, w250, w249) -> (w247:string)
            n119 = Search and Replace String(input string=w247, search string=",", replace string="." ("replace string (\"\")")) -> (result string=w246:string)  [unwired: 5 in, 3 out]
            n120 = Search and Replace String(input string=w246, search string=",", replace string="." ("replace string (\"\")")) -> (result string=w245:string)  [unwired: 5 in, 3 out]
            n121 = call "Dodanie punktu do listy punkty na podstawie współrzędnych geograficznych.vi"("Nazwa punktu"=w248, "UTM"=w261, "Współrzędne punktu"=w245, "Lista wsp. in"=w263) -> ("Lista wsp. out"=w264:string[][])  [unwired: 7 in]
          }
        }
        n122 = Bundle By Name(cluster=T22 {"Kolor punktów z listy"=0, "Położenie startowe robota"={"Pixel y"=0, "Pixel x"=0}} ("Właściwości punktów z listy"), "Kolor punktów z listy"=w207, "Położenie startowe robota"=w208) -> (w205:T22)
        n123 = control-ref of="Dodaj punkt przed docelowym"() -> (w197:refnum<vi>)
        n124 = control-ref of="Punkt do usunięcia"() -> (w211:refnum<vi>)
        n125 = Array Size(array=w196) -> (size(s)=w203:i32[])
        n126 = Index Array(array=w203, index=0) -> (element=w201:i32)
        n127 = call "Aktualizacja listy z punktami do usunięcia -dane z dwoch kolumn.vi"("Lista współrzędnych"=w196, "Lista z punktami do usunięcia"=w197) -> ()  [unwired: 10 in]
        n128 = call "Aktualizacja listy z punktami do usunięcia -dane z dwoch kolumn.vi"("Lista współrzędnych"=w196, "Lista z punktami do usunięcia"=w211) -> ()  [unwired: 10 in]
        n129 = Decrement(x=w201) -> (x-1=w200:i32)
        n130 = local write "Lista współrzędnych"(w196) -> ()
        n131 = call "Dodanie wskazanego punktu z listy współrzędnych do mapy.vi"("Mapa terenu"=w216, "Rozmiar mapy"=w214, "Długość piksela w metrach"=w212, "Nr punktu"=w200, "Lista współrzędnych"=w196, "Właściwości punktów z listy"=w205) -> ("Mapa z wprowadzonym punktem"=w215:picture)  [unwired: 9 in]
      }
      event "Obsługa punktów.Zaznaczony punkt.Dodaj punkt odl.": Value Change {
        n132 = event-data() -> ()  [unwired: 1 in, 1 out]
        n133 = control-ref of="Punkt do usunięcia"() -> (w284:refnum<vi>)
        n134 = Unbundle By Name(w280) -> ("Dł. px[m]"=w276:dbl, "Wpisane punkty na\nliście współrzędnych"=w279:u32)
        n135 = call "Dodanie zaznaczonego punktu na podstawie odległości.vi"("output array in"=w282, "Pocz. poł."=w271, "Obsługa punktów"=w283, "Parametry odwzorowania Ziemi (WGS84)"=w285, "Ring in"=w284) -> ("output array out"=w265:string[][])  [unwired: 6 in]
        n136 = Unbundle By Name(w271) -> ("Piksele"=w273:cluster{"X":i32, "Y":i32})
        n137 = Bundle By Name(cluster=T22 {"Kolor punktów z listy"=0, "Położenie startowe robota"={"Pixel y"=0, "Pixel x"=0}} ("Właściwości punktów z listy"), "Kolor punktów z listy"=w279, "Położenie startowe robota"=w273) -> (w275:T22)
        n138 = Array Size(array=w265) -> (size(s)=w277:i32[])
        n139 = Index Array(array=w277, index=0) -> (element=w268:i32)
        n140 = Decrement(x=w268) -> (x-1=w267:i32)
        n141 = call "Dodanie wskazanego punktu z listy współrzędnych do mapy.vi"("Mapa terenu"=w274, "Rozmiar mapy"=w269, "Długość piksela w metrach"=w276, "Nr punktu"=w267, "Lista współrzędnych"=w265, "Właściwości punktów z listy"=w275) -> ("Mapa z wprowadzonym punktem"=w272:picture)  [unwired: 9 in]
        n142 = local write "Lista współrzędnych"(w265) -> ()
        n143 = control-ref of="Dodaj punkt przed docelowym"() -> (w266:refnum<vi>)
        n144 = control-ref of="Punkt  startowy"() -> (w270:refnum<vi>)
        n145 = call "Aktualizacja listy z punktami do usunięcia -dane z dwoch kolumn.vi"("Lista współrzędnych"=w265, "Lista z punktami do usunięcia"=w266) -> ()  [unwired: 10 in]
        n146 = call "Aktualizacja listy z punktami do usunięcia -dane z dwoch kolumn.vi"("Lista współrzędnych"=w265, "Lista z punktami do usunięcia"=w270) -> ()  [unwired: 10 in]
      }
      event "Zatwierdz ustalony zakres": Value Change {
        n147 = event-data() -> ()  [unwired: 1 in, 1 out]
        n148 = call "Zatwierdzenie ustalonego zakresu.vi"("Skalowanie in"=w295) -> ("Dł. piksela[m]"=w293:dbl, "Skalowanie out"=w294:T8)  [unwired: 9 in]
        n149 = local write "Skalowanie"(w294) -> ()
        n150 = Bundle By Name(cluster=w292, "Dł. px[m]"=w293) -> (w290:T12)
        n151 = local write "Właściwości mapy"(w290) -> ()
        n152 = call "Przeładowanie punktu startowego i punktów docelowych.vi"("Pocz. poł. startu"=w286, "Rozmiar mapy"=w287, "Lista współrzędnych"=w289, "Właściwości mapy"=w290, "Mapa terenu"=w291) -> ("Mapa z wprowadzonym punktem"=w288:picture)  [unwired: 6 in]
      }
      event "Poł. start. wzgl. bazy": Value Change {
        # "Ostatnie zaznaczone na mapie położenie odpowiada lokalizacji robota na mapie terenu."
        n153 = event-data() -> ()  [unwired: 1 in, 1 out]
        n154 = Unbundle By Name(w300) -> ("GPS"=w296:bool)
        n155 = case shown="True" w296 {
          tunnel: w303 -> [_ w309]
          tunnel: w302 -> [w304 w313]
          tunnel: w301 -> [_ w312]
          tunnel: [w304 w305] -> w299
          tunnel: w298 -> [_ w311]
          tunnel: w297 -> [_ w310]
          frame False {
          }
          frame True {
            # "Położenie startu robota na mapie określane na podstawie danych z GPS"
            n156 = local read "Mouse down"() -> (w308:T16)
            n157 = disable-structure shown="Disabled" {
              frame Disabled {
                n158 = local read "Odczyt GPS"() -> ()  [unwired: 1 out]
              }
              frame Enabled {
              }
            }
            n159 = call "Ustawienie startu względem punktu o znanych współrzędnych.vi"("Parametry odwzorowania\n Ziemi (WGS84)"=w309, "Punkt o znanych współrzędnych (baza)"="Punkt o znanych współrzędnych (X)", "Ost. zazn. punkt [px]"=w308) -> ("Poł. startu. out"=w306:T2)  [unwired: 8 in]
            n160 = call "Przeładowanie punktu startowego i punktów docelowych.vi"("Pocz. poł. startu"=w306, "Rozmiar mapy"=w310, "Lista współrzędnych"=w312, "Właściwości mapy"=w311, "Mapa terenu"=w313) -> ("Mapa z wprowadzonym punktem"=w305:picture)  [unwired: 6 in]
            n161 = local write "Poł. X."(w306) -> ()
          }
        }
      }
      event "Właściwości mapy.Zoom mapy": Value Change {
        n162 = event-data() -> ("NewVal"=w319:sgl)  [unwired: 1 in]
        n163 = local read "Mouse down"() -> (w314:T16)
        n164 = control-ref of="Mapa"() -> (w320:refnum<vi>)
        n165 = call "Centrowanie położenia.vi"("Ostatnie położenie robota"=w314, "Mapa z wprowadzonym punktem"=w320) -> ("Przesunięcie wycentrowane"=w317:T16)  [unwired: 9 in]
        n166 = Negate(x=w317) -> (-x=w316:T16)
        n167 = property on="Mapa" class="Pict"("Origin"=w316) -> ()  [unwired: 2 in, 2 out]
        n168 = Bundle By Name(cluster=w315, "Zoom mapy"=w319, "Przesunięcie mapy"=w316, "Ost. zazn. pkt"=w317) -> (w318:T12)
        n169 = property on="Mapa" class="Pict"("ZoomFactor"=w319) -> ()  [unwired: 2 in, 2 out]
        n170 = local write "Właściwości mapy"(w318) -> ()
      }
      event "Centr. Położenie robota": Value Change {
        n171 = event-data() -> ()  [unwired: 1 in, 1 out]
        n172 = local read "Odległość robota  \nod bazy  [m]"() -> (w325:cluster{"X [m]":dbl, "Y [m]":dbl})
        n173 = Unbundle By Name(w330) -> ("Dł. px[m]"=w329:dbl)
        n174 = Unbundle By Name(w327) -> ("Piksele"=w326:cluster{"X":i32, "Y":i32})
        n175 = in-place {
          in-place-border: w329 -> [w340]
          n176 = in-place-cluster #2(w325) -> ("X [m]"=w339:dbl, "Y [m]"=w338:dbl)
          n177 = Divide(x=w338, y=w340) -> (x/y=w341:dbl)
          n178 = Divide(x=w339, y=w340) -> (x/y=w343:dbl)
          n179 = Negate(x=w341) -> (-x=w342:dbl)
          n180 = in-place-cluster #2("X [m]"=w343, "Y [m]"=w342) -> (w328:cluster{"X [m]":dbl, "Y [m]":dbl})
        }
        n181 = Add(x=w328, y=w326) -> (x+y=w324:cluster{dbl, dbl})
        n182 = call "w zakresie mapy.vi"("Rozmiar mapy"=w323, "Poł. piksel"=w324) -> ("Boolean"=w322:bool)  [unwired: 9 in]
        n183 = case shown="True" w322 {
          tunnel: w330 -> [_ w333]
          tunnel: w324 -> [_ w332]
          frame False {
          }
          frame True {
            n184 = control-ref of="Mapa"() -> (w337:refnum<vi>)
            n185 = call "Centrowanie położenia.vi"("Ostatnie położenie robota"=w332, "Mapa z wprowadzonym punktem"=w337) -> ("Przesunięcie wycentrowane"=w335:T16)  [unwired: 9 in]
            n186 = Negate(x=w335) -> (-x=w334:T16)
            n187 = Bundle By Name(cluster=w333, "Przesunięcie mapy"=w334, "Ost. zazn. pkt"=w335) -> (w336:T12)
            n188 = property on="Mapa" class="Pict"("Origin"=w334) -> ()  [unwired: 2 in, 2 out]
            n189 = local write "Właściwości mapy"(w336) -> ()
          }
        }
      }
      event "Poł. start. robota": Value Change {
        # "Po wyborze poł. start. robota ostatni zaznaczony punkt na mapie staje się położenia m startowym."
        n190 = event-data() -> ()  [unwired: 1 in, 1 out]
        n191 = Unbundle By Name(w354) -> ("GPS"=w353:bool)
        n192 = Unbundle By Name(w351) -> ("Ost. zazn. pkt"=w349:cluster{"X":i32, "Y":i32})
        n193 = call "w zakresie mapy.vi"("Rozmiar mapy"=w350, "Poł. piksel"=w349) -> ("Boolean"=w348:bool)  [unwired: 9 in]
        n194 = Bundle By Name(cluster=w344, "Piksele"=w349) -> (w345:T2)
        n195 = Select(t=w345, s=w348, f=w344) -> (s? t:f=w347:T2)
        n196 = case shown="True" w353 {
          tunnel: w347 -> [w357 w359]
          tunnel: [w357 w358] -> w346
          frame False {
            # "Zapisanie do położenia startowego lokalizacji startu w pikselach bez uwzględnienia położenia GPS."
          }
          frame True {
            # "Zapisanie do położenia startowego lokalizacji startu w pikselach oraz dane GPS dla tego punktu."
            n197 = local read "Odczyt GPS"() -> (w361:T14)
            n198 = Unbundle By Name(w361) -> ("Położenie \nrobota  UTM"=w360:T28)
            n199 = Bundle By Name(cluster=w359, "UTM"=w360) -> (w358:T2)
          }
        }
        n200 = call "Przeładowanie punktu startowego i punktów docelowych.vi"("Pocz. poł. startu"=w346, "Rozmiar mapy"=w350, "Lista współrzędnych"=w356, "Właściwości mapy"=w351, "Mapa terenu"=w355) -> ("Mapa z wprowadzonym punktem"=w352:picture)  [unwired: 6 in]
        n201 = local write "Poł. X."(w346) -> ()
      }
      event "stop": Value Change {
        w366 = 0.0 ("V_postepowa")
        n202 = event-data() -> ()  [unwired: 1 in, 1 out]
        n203 = Bundle By Name(cluster=w369, "Przesunięcie mapy"=T23 {"Horizontal"=0, "Vertical"=0} ("Origin")) -> (w368:T12)
        n204 = shared-variable "My Computer\\Biblioteka moduł map v3.lvlib\\Zmienne.lvlib\\Predkosci robota.lvlib\\V_postepowa"(w366) -> ()  [unwired: 1 in, 1 out]
        n205 = shared-variable "My Computer\\Biblioteka moduł map v3.lvlib\\Zmienne.lvlib\\Predkosci robota.lvlib\\w-obrotowa"(w366) -> ()  [unwired: 1 in, 1 out]
        n206 = local write "Właściwości mapy"(w368) -> ()
        n207 = Two Button Dialog(message="Czy zakończyć działanie programu?", 1:"NIE" ("F button name (\"Cancel\")"), 2:"TAK" ("T button name (\"OK\")")) -> (T button?=w365:bool)
        n208 = Send Notification(notification=w365, notifier=w370) -> ()  [unwired: 1 in, 2 out]
      }
      event "Mapa": Mouse Down {
        # "Odczyt lokalizacji kursora po kliknięciu na mapie."
        n209 = event-data() -> ()  [unwired: 1 in, 2 out]
        n210 = property on="Mapa" class="Pict"() -> ("Mouse"=w373:T25)  [unwired: 2 in, 2 out]
        n211 = Unbundle By Name(w373) -> ("Mouse Position"=w372:cluster{"X":i32, "Y":i32})
        n212 = local write "Mouse down"(w372) -> ()
      }
      event "Mapa": Mouse Up {
        # "Wyznaczenie zmiany położenia przed i po kliknięciu."
        n213 = event-data() -> ()  [unwired: 1 in, 1 out]
        n214 = property on="Mapa" class="Pict"() -> ("Mouse"=w385:T25)  [unwired: 2 in, 2 out]
        n215 = call "Ustalenie nowego przesunięcia mapy po mose down-up.vi"("Właściwości mapy in"=w386, "Pocz. poł."=w375, "Obsługa punktów in"=w384, "Mouse down \ncoords"="Mouse down", "Mouse"=w385) -> ("Właściwości mapy out"=w381:T26, "Obsługa punktów out"=w383:T27)  [unwired: 5 in]
        n216 = local write "Obsługa punktów"(w383) -> ()
        n217 = local write "Właściwości mapy"(w381) -> ()
        n218 = Unbundle By Name(w381) -> ("Ost. zazn. pkt."=w376:cluster{"X":i32, "Y":i32}, "Przesunięcie mapy"=w380:cluster{"X":i16, "Y":i16})
        n219 = Unbundle By Name(w377) -> ("Wybór \nznacznika"=w379:bool, "Blokada \nznaczników"=w378:bool)
        n220 = property on="Mapa" class="Pict"("Origin"=w380) -> ()  [unwired: 2 in, 2 out]
        n221 = case shown="False" w378 {
          tunnel: w379 -> [w391 _]
          tunnel: w377 -> [w390 _]
          tunnel: w376 -> [w388 _]
          frame False {
            n222 = case shown="True" w391 {
              tunnel: w390 -> [w394 w397]
              tunnel: [w393 w396] -> w389
              tunnel: w388 -> [w392 w395]
              frame False {
                n223 = Bundle By Name(cluster=w394, "Polozenie 1"=w392) -> (w393:T8)
              }
              frame True {
                n224 = Bundle By Name(cluster=w397, "Polozenie 2"=w395) -> (w396:T8)
              }
            }
            n225 = local write "Skalowanie"(w389) -> ()
          }
          frame True {
          }
        }
      }
      event "Wpr. pkt. wsp. z pliku": Value Change {
        n226 = event-data() -> ()  [unwired: 1 in, 1 out]
        n227 = Unbundle By Name(w403) -> ("UTM"=w407:T24)
        n228 = call-poly <vilib>:"Read From Spreadsheet File.vi"("file path (dialog if empty)"="Plik z punktami wsp. geograficzne") -> ("all rows"=w406:string[][])  [unwired: 6 in, 4 out]
        n229 = Array Size(array=w406) -> (size(s)=w411:i32[])
        n230 = Index Array(array=w411, index=0) -> (element=w409:i32)
        n231 = for {
          N: w409 -> [_]
          shift-right: [w422] -> w398
          shift-left: w408 -> [w420]
          tunnel: w407 -> [w421]
          tunnel: w406 -> [w419] mode=indexing
          tunnel: w406 -> [w418] mode=indexing
          n232 = Index Array(array=w418, index=0) -> (element=w414:string)
          n233 = Index Array(array=w419, index=1) -> (element=w415:string)
          n234 = call "Dodanie punktu do listy punkty na podstawie współrzędnych geograficznych.vi"("Nazwa punktu"=w414, "UTM"=w421, "Współrzędne punktu"=w415, "Lista wsp. in"=w420) -> ("Lista wsp. out"=w422:string[][])  [unwired: 7 in]
        }
        n235 = local write "Lista współrzędnych"(w398) -> ()
        n236 = call "Przeładowanie punktu startowego i punktów docelowych.vi"("Pocz. poł. startu"=w403, "Rozmiar mapy"=w400, "Lista współrzędnych"=w398, "Właściwości mapy"=w404, "Mapa terenu"=w401) -> ("Mapa z wprowadzonym punktem"=w405:picture)  [unwired: 6 in]
        n237 = control-ref of="Punkt do usunięcia"() -> (w413:refnum<vi>)
        n238 = control-ref of="Dodaj punkt przed docelowym"() -> (w399:refnum<vi>)
        n239 = control-ref of="Punkt  startowy"() -> (w402:refnum<vi>)
        n240 = call "Aktualizacja listy z punktami do usunięcia -dane z dwoch kolumn.vi"("Lista współrzędnych"=w398, "Lista z punktami do usunięcia"=w413) -> ()  [unwired: 10 in]
        n241 = call "Aktualizacja listy z punktami do usunięcia -dane z dwoch kolumn.vi"("Lista współrzędnych"=w398, "Lista z punktami do usunięcia"=w402) -> ()  [unwired: 10 in]
        n242 = call "Aktualizacja listy z punktami do usunięcia -dane z dwoch kolumn.vi"("Lista współrzędnych"=w398, "Lista z punktami do usunięcia"=w399) -> ()  [unwired: 10 in]
      }
      event "Obsługa punktów.Zaznaczony punkt.Odl. do pkt [m]": Value Change {
        n243 = event-data() -> ()  [unwired: 1 in, 1 out]
        n244 = Unbundle By Name(w423) -> ("Piksele.X"=w432:i32, "Piksele.Y"=w431:i32)
        n245 = Unbundle By Name(w430) -> ("Dł. px[m]"=w436:dbl)
        n246 = Unbundle By Name(w426) -> ("Zaznaczony punkt.Odl. do pkt [m].X"=w425:dbl, "Zaznaczony punkt.Odl. do pkt [m].Y"=w424:dbl)
        n247 = Divide(x=w425, y=w436) -> (x/y=w434:dbl)
        n248 = Negate(x=w424) -> (-x=w435:dbl)
        n249 = Divide(x=w435, y=w436) -> (x/y=w433:dbl)
        n250 = Add(x=w434, y=w432) -> (x+y=w429:dbl)
        n251 = Add(x=w433, y=w431) -> (x+y=w428:dbl)
        n252 = Bundle By Name(cluster=w430, "Ost. zazn. pkt.X"=w429, "Ost. zazn. pkt.Y"=w428) -> (w427:T12)
        n253 = local write "Właściwości mapy"(w427) -> ()
      }
      event "Obsługa punktów.Wsp. geograficzne.Dodaj punkt wsp.": Value Change {
        n254 = event-data() -> ()  [unwired: 1 in, 1 out]
        n255 = Unbundle By Name(w442) -> ("UTM"=w458:T24)
        n256 = Unbundle By Name(w455) -> ("Wsp. geograficzne.Nazwa"=w457:string, "Wsp. geograficzne.Współrzędna punktu"=w456:string)
        n257 = Unbundle By Name(w451) -> ("Dł. px[m]"=w448:dbl, "Wpisane punkty na\nliście współrzędnych"=w453:u32)
        n258 = Unbundle By Name(w442) -> ("Piksele"=w452:cluster{"X":i32, "Y":i32})
        n259 = Bundle By Name(cluster=T22 {"Kolor punktów z listy"=0, "Położenie startowe robota"={"Pixel y"=0, "Pixel x"=0}} ("Właściwości punktów z listy"), "Kolor punktów z listy"=w453, "Położenie startowe robota"=w452) -> (w447:T22)
        n260 = call "Dodanie punktu do listy punkty na podstawie współrzędnych geograficznych.vi"("Nazwa punktu"=w457, "UTM"=w458, "Współrzędne punktu"=w456, "Lista wsp. in"=w460) -> ("Lista wsp. out"=w438:string[][])  [unwired: 7 in]
        n261 = control-ref of="Punkt do usunięcia"() -> (w459:refnum<vi>)
        n262 = call "Aktualizacja listy z punktami do usunięcia -dane z dwoch kolumn.vi"("Lista współrzędnych"=w438, "Lista z punktami do usunięcia"=w459) -> ()  [unwired: 10 in]
        n263 = control-ref of="Dodaj punkt przed docelowym"() -> (w439:refnum<vi>)
        n264 = Array Size(array=w438) -> (size(s)=w449:i32[])
        n265 = control-ref of="Punkt  startowy"() -> (w441:refnum<vi>)
        n266 = local write "Lista współrzędnych"(w438) -> ()
        n267 = Index Array(array=w449, index=0) -> (element=w445:i32)
        n268 = call "Aktualizacja listy z punktami do usunięcia -dane z dwoch kolumn.vi"("Lista współrzędnych"=w438, "Lista z punktami do usunięcia"=w439) -> ()  [unwired: 10 in]
        n269 = call "Aktualizacja listy z punktami do usunięcia -dane z dwoch kolumn.vi"("Lista współrzędnych"=w438, "Lista z punktami do usunięcia"=w441) -> ()  [unwired: 10 in]
        n270 = Decrement(x=w445) -> (x-1=w444:i32)
        n271 = call "Dodanie wskazanego punktu z listy współrzędnych do mapy.vi"("Mapa terenu"=w446, "Rozmiar mapy"=w440, "Długość piksela w metrach"=w448, "Nr punktu"=w444, "Lista współrzędnych"=w438, "Właściwości punktów z listy"=w447) -> ("Mapa z wprowadzonym punktem"=w443:picture)  [unwired: 9 in]
      }
    }
  }
  n272 = while "Pętla sterowania robota" {
    tunnel: w1 -> [w489]
    shift-right: [w484] -> _
    shift-left: T17."Pobranie punktu" -> [w487]
    shift-right: [w485] -> _
    shift-left: w14 -> [w486]
    tunnel: "Parametry odwzorowania\n Ziemi (WGS84)" -> [w475]
    tunnel: "Ustawienia początkowe" -> [w474]
    tunnel: "Azymut robota\n pocz/nowy" -> [w476]
    tunnel: "Ustawienia początkowe" -> [w481]
    i -> [w482]
    stop <- w488 stop-if-true
    # "Odbiór danych z robota i określanie jego położenia względem punktu startowego"
    n273 = Get Notifier Status(notifier=w489) -> (current notification=w488:bool)  [unwired: 1 in, 4 out]
    n274 = local read "Poł. X."() -> (w473:T2)
    n275 = Wait Until Next ms Multiple(millisecond multiple=u32 50) -> ()  [unwired: 1 out]
    n276 = call "Analiza położeń robotów.vi"("Zapis danych z przejazdu"="Zapis danych z przejazdu", "Azymut łazika\n pocz/nowy"=w476, "Parametry odwzorowania\n Ziemi (WGS84)"=w475, "Ustawienia początkowe"=w474, "Poł. bazy."=w473, "Wybór robota"="Wybór robota", "Reset"="Reset") -> ("Azymut"=→"Azymut":dbl, "Odległość robota od bazy  [m]"=w469:cluster{"X [m]":dbl, "Y [m]":dbl}, "Lokalizacja robotów"=w466:T1, "Odczyt GPS - Łazik 2"=→"Odczyt GPS":T14)  [unwired: 5 in]
    "Lokalizacja robotów 2" <- w466
    "Odległość robota  \nod bazy  [m]" <- w469
    n277 = local read "Lista współrzędnych"() -> (w463:string[][])
    n278 = call "Odległośc pomiędzy wybranymi robotami.vi"("Lokalizacja robotów in"=w466, "Wybór robota 2"="Wybór robota 3", "Wybór robota in"="Wybór robota 2") -> ("Odległość pomiędzy\n robotami [m]"=→"Odległość pomiędzy\n robotami [m]":dbl, "Odległości pomiędzy wybranymi robotami xy [m]"=→"Odległości pomiędzy wybranymi robotami xy [m]":cluster{"X [m]":dbl, "Y [m]":dbl})  [unwired: 7 in]
    n279 = call "Aktualizacja odległości.vi"("Odległośćrobota od startu [m]"=w469, "Lista współrzędnych"=w463) -> ("Lista współrzędnych 2"=w464:string[][])  [unwired: 9 in]
    "Lista współrzędnych" <- w464
    n280 = property on="Lokalizacja robotów 2" class="Clust (strict)"("Visible"=FALSE) -> ()  [unwired: 2 in, 2 out]
    n281 = case shown="True" "jazda" {
      tunnel: w487 -> [_ w518]
      tunnel: w486 -> [_ w515]
      tunnel: [w490 w517] -> w485
      tunnel: [T17."Obrót i dojazd do punktu" w516] -> w484
      tunnel: w482 -> [_ w505]
      tunnel: w481 -> [_ w504]
      tunnel: w464 -> [_ w503]
      tunnel: "Dodaj punkt przed docelowym" -> [_ w502]
      frame False {
        w492 = 0.0 ("V_postepowa")
        n282 = global write "V - prędkość postępowa.vi" "V - prędkość postępowa"(0.0 ("V - prędkość postępowa")) -> ()
        n283 = global write "w - prękdość kątowa.vi" "w - prędkość kątowa"(0.0 ("w - prędkość kątowa")) -> ()
        n284 = shared-variable "My Computer\\Biblioteka moduł map v3.lvlib\\Zmienne.lvlib\\Predkosci robota.lvlib\\V_postepowa"(w492) -> ()  [unwired: 1 in, 1 out]
        n285 = shared-variable "My Computer\\Biblioteka moduł map v3.lvlib\\Zmienne.lvlib\\Predkosci robota.lvlib\\w-obrotowa"(w492) -> ()  [unwired: 1 in, 1 out]
        n286 = local read "Punkt  startowy"() -> (w491:u16)
        n287 = Decrement(x=w491) -> (x-1=w490:u16)
      }
      frame True {
        n288 = call "Pobranie odległości do punktu docelowego z listy współrzędnych.vi"("Lista współrzędnych"=w503, "Numer pobranego punktu"=w515) -> ("Kąt trygonometryczny skierowany od położenia robota na pkt. docelowy [radiany]"=w514:dbl, "Odległość do punktu"=w513:dbl, "Dojazd do punktu"=w509:string, "Odl. pkt. od startu"=→"Odl. pkt. od startu":cluster{"E/x[m]":dbl, "N/y[m]":dbl})  [unwired: 6 in]
        "Punkt\n docelowy" <- w509
        n289 = To Lower Case(string=w509) -> (all lower case string=w511:string)
        n290 = xnode "Match Regular Expression"("input string"=w511, "regular expression"="p") -> ("whole match"=w508:string)  [unwired: 4 in, 4 out]
        n291 = Empty String/Path?(string/path=w508) -> (empty?=w500:bool)
        n292 = Select(t="zad. promien \nodlegl. [m]", s=w500, f=2.0 ("t")) -> (s? t:f=w501:dbl)
        n293 = Greater Or Equal?(x=w501, y=w513) -> (x >= y?=w507:bool)
        n294 = And(x=w507, y=w500) -> (x .and. y?=→"Osiągnięcie punktu":bool)
        n295 = case shown="False" "2. Autonomia" {
          tunnel: [T17."Obrót i dojazd do punktu" w650] -> w516
          tunnel: w518 -> [_ w651]
          tunnel: [w634 w649] -> w517
          tunnel: w515 -> [_ w648]
          tunnel: w514 -> [_ w647]
          tunnel: w513 -> [_ w646]
          tunnel: w507 -> [_ w645]
          tunnel: w505 -> [_ w644]
          tunnel: [0.0 ("y") w643] -> w496
          tunnel: [0.0 ("w - prędkość kątowa") w642] -> w497
          tunnel: w509 -> [_ w641]
          tunnel: w504 -> [_ w640]
          tunnel: w503 -> [_ w639]
          tunnel: w502 -> [_ _]
          frame False {
            n296 = Decrement(x="Punkt  startowy") -> (x-1=w634:u16)
          }
          frame True {
            n297 = case shown="\"Pobranie punktu\", Default" w651 {
              tunnel: [T17."Obrót i dojazd do punktu" w678 w694] -> w650
              tunnel: w648 -> [w654 w676 w693]
              tunnel: [w652 w676 w693] -> w649
              tunnel: w647 -> [_ w675 _]
              tunnel: w646 -> [_ w674 _]
              tunnel: [_ w668 _] -> w643
              tunnel: [_ w664 _] -> w642
              tunnel: w645 -> [_ w672 _]
              tunnel: w644 -> [w660 w671 _]
              tunnel: w641 -> [_ _ w687]
              tunnel: w640 -> [_ w663 _]
              tunnel: w639 -> [w659 _ _]
              frame "Pobranie punktu", Default {
                n298 = Array Size(array=w659) -> (size(s)=w658:i32[])
                n299 = Index Array(array=w658, index=0) -> (element=w656:i32)
                n300 = Greater Or Equal?(x=w654, y=w656) -> (x >= y?=w655:bool)
                n301 = Increment(x=w654) -> (x+1=w653:i32)
                n302 = Select(t=w654, s=w655, f=w653) -> (s? t:f=w652:i32)
                "Numeric" <- w660
              }
              frame "Obrót i dojazd do punktu" {
                w667 = 25.0 ("input variable")
                n303 = property on="Numeric" class="DigNum (strict)"() -> ("Value"=w670:i32)  [unwired: 2 in, 2 out]
                n304 = Unbundle By Name(w663) -> ("Dane z"=w662:bool)
                n305 = Subtract(x=w671, y=w670) -> (x-y=w666:i32)
                n306 = call "Regulator.vi"("Odczyt odom"=w662, "Parametry regulatora"="Parametry regulatora", "Odległość do punktu"=w674, "Kąt tryg. zad"=w675) -> ("w - prędkość kątowa"=w665:dbl, "V - prędkość postępowa"=w669:dbl)  [unwired: 6 in]
                n307 = Get Date/Time In Seconds() -> (seconds since 1Jan1904=→"Obr. doj. do pkt.":timestamp)
                n308 = formula code="if(i<T)\ny=x*i/T;\nelse\ny=x;"("x"=w665, "i"=w666, "T"=w667) -> ("y"=w664:dbl)
                n309 = formula code="if(i<T)\ny=x*i/T;\nelse\ny=x;"("x"=w669, "i"=w666, "T"=w667) -> ("y"=w668:dbl)
                n310 = Select(t=T17."Zatrzymanie w punkcie", s=w672, f=T17."Obrót i dojazd do punktu") -> (s? t:f=w678:T17)
              }
              frame "Zatrzymanie w punkcie" {
                # "jest p"
                n311 = local read "Obr. doj. do pkt."() -> (w698:timestamp)
                n312 = To Lower Case(string=w687) -> (all lower case string=w688:string)
                n313 = Get Date/Time In Seconds() -> (seconds since 1Jan1904=w697:timestamp)
                n314 = xnode "Match Regular Expression"("input string"=w688, "regular expression"="p") -> ("whole match"=w685:string)  [unwired: 4 in, 4 out]
                n315 = Subtract(x=w697, y=w698) -> (x-y=w699:dbl)
                n316 = Greater Or Equal?(x=w699, y="Time to wait [s]") -> (x >= y?=w691:bool)
                n317 = Empty String/Path?(string/path=w685) -> (empty?=w684:bool)
                n318 = Not(x=w684) -> (.not. x?=w683:bool)
                n319 = Select(t=w691, s="button/time", f="go forward") -> (s? t:f=w682:bool)
                n320 = Or(x=w683, y=w682) -> (x .or. y?=w681:bool)
                n321 = Select(t=T17."Pobranie punktu", s=w681, f=T17."Zatrzymanie w punkcie") -> (s? t:f=w694:T17)
              }
            }
          }
        }
        "V - prędkość postępowa" <- w496
        "w - prędkość kątowa" <- w497
        n322 = shared-variable "My Computer\\Biblioteka moduł map v3.lvlib\\Zmienne.lvlib\\Predkosci robota.lvlib\\w-obrotowa"(w497) -> ()  [unwired: 1 in, 1 out]
        n323 = global write "w - prękdość kątowa.vi" "w - prędkość kątowa"(w497) -> ()
        n324 = global write "V - prędkość postępowa.vi" "V - prędkość postępowa"(w496) -> ()
        n325 = shared-variable "My Computer\\Biblioteka moduł map v3.lvlib\\Zmienne.lvlib\\Predkosci robota.lvlib\\V_postepowa"(w496) -> ()  [unwired: 1 in, 1 out]
      }
    }
  }
